vi "limits.vi"(2 "ON":bool, 3 "STATE":T1, 4 "CONN":bool, 5 "ALR code":T2=enum."H") -> (1 "LIMIT":bool)   [LabVIEW 2019, in "Alarms.lvlib"]
uses:
  Alarms.lvlib
  Ctl/ALR code.ctl
  Inputs/Ctl/Parameter State.ctl
  Inputs/Inputs.lvlib
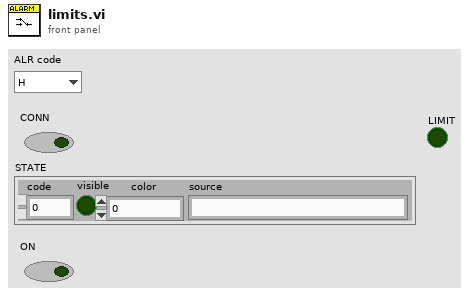
[diagram p1: front panel]
types:
  T1 = typedef "Inputs.lvlib/Parameter State.ctl" = cluster{"code":i32, "visible":bool, "color":u32, "source":string}
  T2 = typedef "Alarms.lvlib/ALR code.ctl" = enum16{"CONN", "H", "HH", "L", "LL", "SERR", "ON", "OFF", "XM19", "XM24", "XM47", "XM51", "XM52", "XM53", "XM54", "XM55", "XM56", "XM61", "XM62", "XM63", "XM64", "XM65", "XM66"}
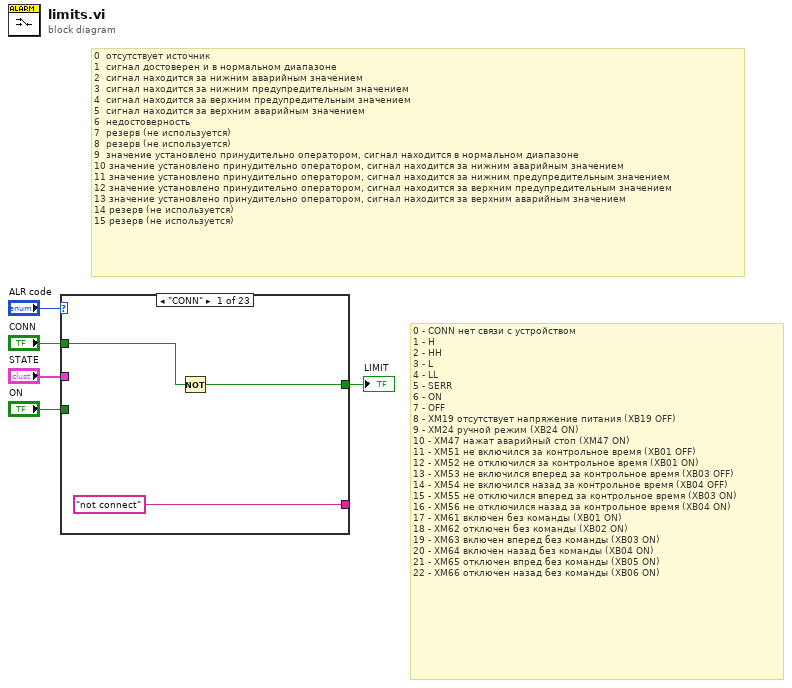
[diagram p0: block diagram]
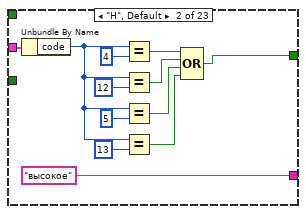
[diagram p2: hidden frame]
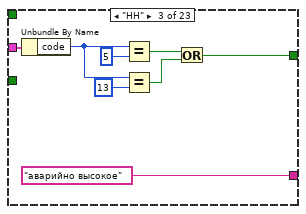
[diagram p3: hidden frame]
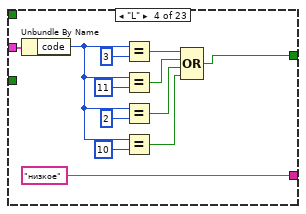
[diagram p4: hidden frame]
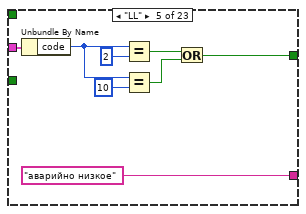
[diagram p5: hidden frame]
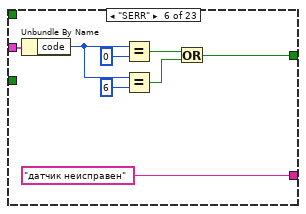
[diagram p6: hidden frame]
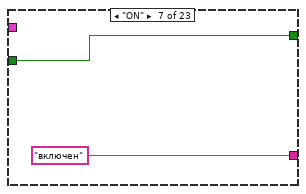
[diagram p7: hidden frame]
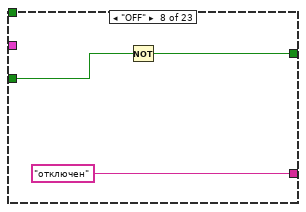
[diagram p8: hidden frame]
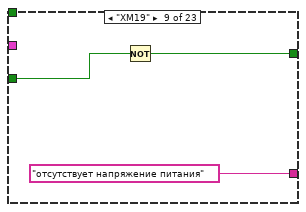
[diagram p9: hidden frame]
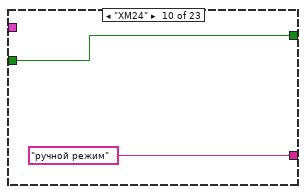
[diagram p10: hidden frame]
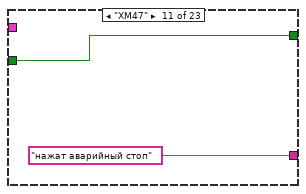
[diagram p11: hidden frame]
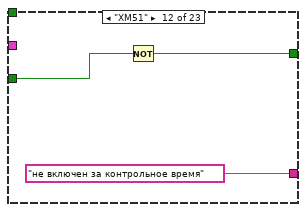
[diagram p12: hidden frame]
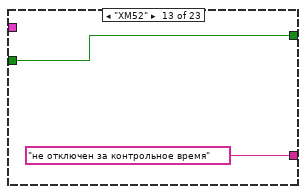
[diagram p13: hidden frame]
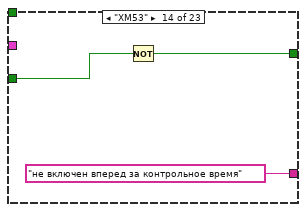
[diagram p14: hidden frame]
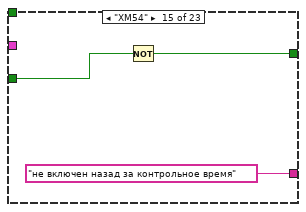
[diagram p15: hidden frame]
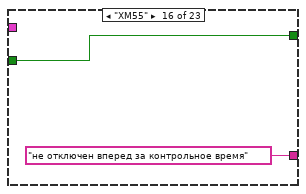
[diagram p16: hidden frame]
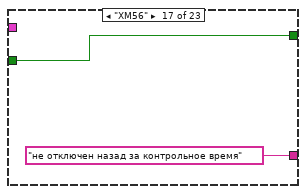
[diagram p17: hidden frame]
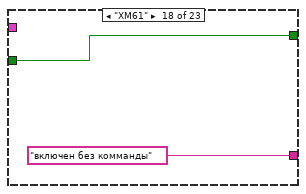
[diagram p18: hidden frame]
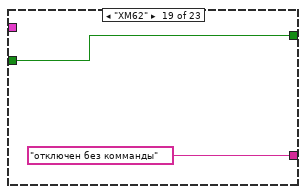
[diagram p19: hidden frame]
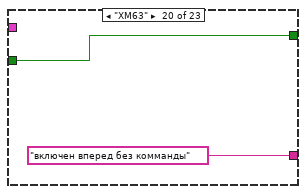
[diagram p20: hidden frame]
diagram:
  # "0 - CONN нет связи с устройством\n1 - H\n2 - HH\n3 - L\n4 - LL\n5 - SERR\n6 - ON\n7 - OFF\n8 - XM19\tотсутствует напряжение питания (XB19 OFF)\n9 - XM24\tручной режим (XB24 ON)\n10 - XM47\tнажат аварийный стоп (XМ47 ON)\n11 - XM51\tне включился за контрольное время (XB01 OFF)\n12 - XM52\tне отключился за контрольное время (XB01 ON)\n13 - XM53\tне включился вперед за контрольное время (XB03 OFF)\n14 - XM54\tне включился назад за контрольное время (XB04 OFF)\n15 - XM55\tне отключился вперед за контрольное время (XB03 ON)\n16 - XM56\tне отключился назад за контрольное время (XB04 ON)\n17 - XM61\tвключен без команды (XB01 ON)\n18 - XM62\tотключен без команды (XB02 ON)\n19 - XM63\tвключен вперед без команды (XB03 ON)\n20 - XM64\tвключен назад без команды (XB04 ON)\n21 - XM65\tотключен впред без команды (XB05 ON)\n22 - XM66\tотключен назад без команды (XB06 ON)"
  # "0  отсутствует источник\n1  сигнал достоверен и в нормальном диапазоне\n2  сигнал находится за нижним аварийным значением\n3  сигнал находится за нижним предупредительным значением\n4  сигнал находится за верхним предупредительным значением\n5  сигнал находится за верхним аварийным значением\n6  недостоверность\n7  резерв (не используется)\n8  резерв (не используется)\n9  значение установлено принудительно оператором, сигнал находится в нормальном диапазоне\n10 значение установлено принудительно оператором, сигнал находится за нижним аварийным значением\n11 значение установлено принудительно оператором, сигнал находится за нижним предупредительным значением\n12 значение установлено принудительно оператором, сигнал находится за верхним предупредительным значением\n13 значение установлено принудительно оператором, сигнал находится за верхним аварийным значением\n14 резерв (не используется)\n15 резерв (не используется)"
  n1 = case shown="\"CONN\"" "ALR code" {
    tunnel: "STATE" -> [_ w20 w28 w40 w48 w56 _ _ _ _ _ _ _ _ _ _ _ _ _ _ _ _ _]
    tunnel: [w7 w15 w22 w35 w42 w50 w57 w59 w62 w65 w67 w69 w72 w74 w77 w80 w82 w84 w86 w88 w90 w92 w94] -> w5
    tunnel: ["not connect" ("source") "высокое" ("source") "аварийно высокое" ("source") "низкое" ("source") "аварийно низкое" ("source") "датчик неисправен" ("source") "включен" ("source") "отключен" ("source") "отсутствует напряжение питания" ("source") "ручной режим" ("source") "нажат аварийный стоп" ("source") "не включен за контрольное время" ("source") "не отключен за контрольное время" ("source") "не включен вперед за контрольное время" ("source") "не включен назад за контрольное время" ("source") "не отключен вперед за контрольное время" ("source") "не отключен назад за контрольное время" ("source") "включен без комманды" ("source") "отключен без комманды" ("source") "включен вперед без комманды" ("source") "включен назад без комманды" ("source") "отключен вперед без комманды" ("source") "отключен назад без комманды" ("source")] -> _
    tunnel: "ON" -> [_ _ _ _ _ _ w57 w60 w63 w65 w67 w70 w72 w75 w78 w80 w82 w84 w86 w88 w90 w92 w94]
    tunnel: "CONN" -> [w6 _ _ _ _ _ _ _ _ _ _ _ _ _ _ _ _ _ _ _ _ _ _]
    frame "CONN" {
      n2 = Not(x=w6) -> (.not. x?=w7:bool)
    }
    frame "H", Default {
      n3 = Unbundle By Name(w20) -> ("code"=w12:i32)
      n4 = Equal?(x=w12, y=4) -> (x = y?=w17:bool)
      n5 = Equal?(x=w12, y=12) -> (x = y?=w16:bool)
      n6 = Equal?(x=w12, y=5) -> (x = y?=w11:bool)
      n7 = Equal?(x=w12, y=13) -> (x = y?=w10:bool)
      n8 = Compound Arithmetic op=OR(w17, w16, w11, w10) -> (w15:bool)
    }
    frame "HH" {
      n9 = Unbundle By Name(w28) -> ("code"=w25:i32)
      n10 = Equal?(x=w25, y=5) -> (x = y?=w24:bool)
      n11 = Equal?(x=w25, y=13) -> (x = y?=w23:bool)
      n12 = Or(x=w24, y=w23) -> (x .or. y?=w22:bool)
    }
    frame "L" {
      n13 = Unbundle By Name(w40) -> ("code"=w32:i32)
      n14 = Equal?(x=w32, y=3) -> (x = y?=w37:bool)
      n15 = Equal?(x=w32, y=11) -> (x = y?=w36:bool)
      n16 = Equal?(x=w32, y=2) -> (x = y?=w31:bool)
      n17 = Equal?(x=w32, y=10) -> (x = y?=w30:bool)
      n18 = Compound Arithmetic op=OR(w37, w36, w31, w30) -> (w35:bool)
    }
    frame "LL" {
      n19 = Unbundle By Name(w48) -> ("code"=w45:i32)
      n20 = Equal?(x=w45, y=2) -> (x = y?=w44:bool)
      n21 = Equal?(x=w45, y=10) -> (x = y?=w43:bool)
      n22 = Or(x=w44, y=w43) -> (x .or. y?=w42:bool)
    }
    frame "SERR" {
      n23 = Unbundle By Name(w56) -> ("code"=w53:i32)
      n24 = Equal?(x=w53, y=0) -> (x = y?=w52:bool)
      n25 = Equal?(x=w53, y=6) -> (x = y?=w51:bool)
      n26 = Or(x=w52, y=w51) -> (x .or. y?=w50:bool)
    }
    frame "ON" {
    }
    frame "OFF" {
      n27 = Not(x=w60) -> (.not. x?=w59:bool)
    }
    frame "XM19" {
      n28 = Not(x=w63) -> (.not. x?=w62:bool)
    }
    frame "XM24" {
    }
    frame "XM47" {
    }
    frame "XM51" {
      n29 = Not(x=w70) -> (.not. x?=w69:bool)
    }
    frame "XM52" {
    }
    frame "XM53" {
      n30 = Not(x=w75) -> (.not. x?=w74:bool)
    }
    frame "XM54" {
      n31 = Not(x=w78) -> (.not. x?=w77:bool)
    }
    frame "XM55" {
    }
    frame "XM56" {
    }
    frame "XM61" {
    }
    frame "XM62" {
    }
    frame "XM63" {
    }
    frame "XM64" {
    }
    frame "XM65" {
    }
    frame "XM66" {
    }
  }
  "LIMIT" <- w5
